vi "读取Function.vi"(8 "error in (no error)":errorcluster caption="错误输入（无错误）", 11 "DMM输入":refnum<class "DMM.lvclass">) -> (0 "error out":errorcluster caption="错误输出", 2 "Function":T1(ring), 3 "DMM输出":refnum<class "DMM.lvclass">)   [LabVIEW 2020, in "DMM.lvlib" / "DMM.lvclass"]
uses:
  DMM.lvclass
  DMM.lvclass/DMM.ctl
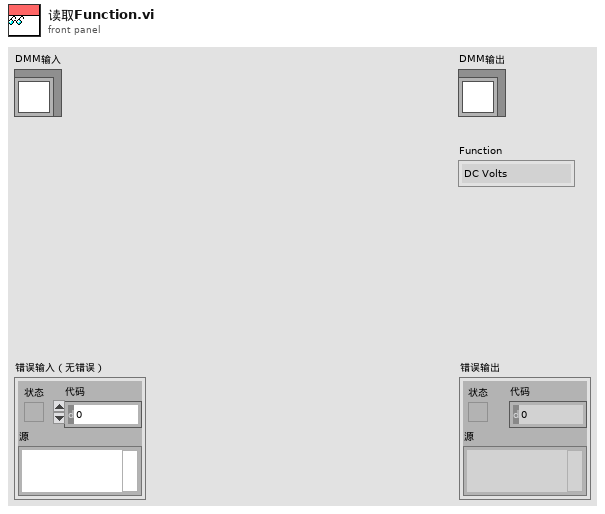
[diagram p1: front panel]
types:
  T1 = enum16{"DC Volts", "AC Volts", "DC Current", "AC Current", "2-Wire Resistance", "4-Wire Resistance"}
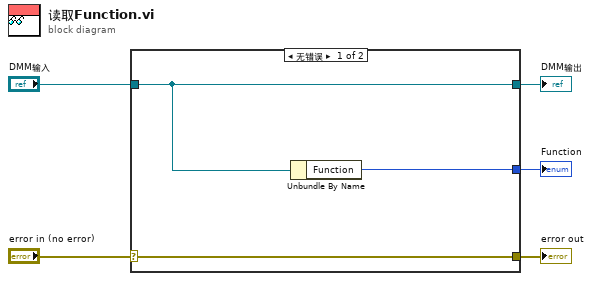
[diagram p0: block diagram]
diagram:
  n1 = case shown="无错误" "error in (no error)" {
    selector: "error in (no error)" -> [w8 w9]
    tunnel: [w8 w9] -> w4
    tunnel: [w7 w10] -> w2
    tunnel: "DMM输入" -> [w7 w10]
    tunnel: [w6 _] -> w1
    frame No Error {
      n2 = Unbundle By Name(w7) -> ("Function"=w6:T1)
    }
    frame Error {
    }
  }
  "error out" <- w4
  "DMM输出" <- w2
  "Function" <- w1
